vi "Test Harness.vi"(9 "Solver VI":refnum<vi>, 10 "Word List":string[](array[string])=["YELLOW", "ORANGE", "PURPLE", "BLUE", "GREEN", "RED"], 11 "Word Search Grid":string[][](array[string])=[["R", "B", "L", "U", "E", "W"], ["E", "G", "N", "A", "R", "O"], ["D", "B", "C", "E", "W", "L"], ["L", "L", "D", "K", "V", "L"], ["P", "U", "R", "P", "L", "E"], ["N", "E", "E", "R", "G", "Y"]]) -> (2 "All Words Found":bool, 3 "Execution Time":dbl)   [LabVIEW 2024]
panel:
  # "Use this Test Harness VI to time your Word Search solution (and ensure it works correctly)."
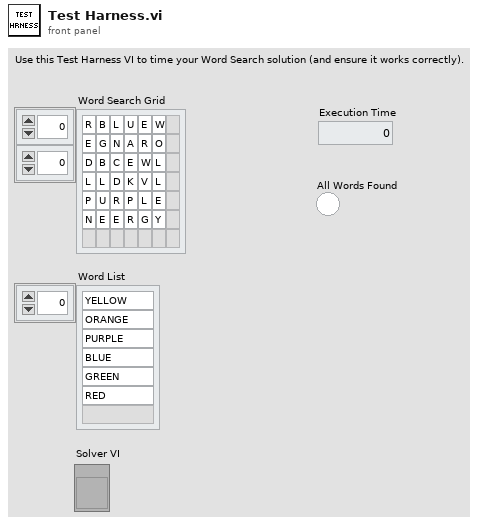
[diagram p1: front panel]
types:
  T1 = typedef "Word Search Scorer.lvlib/Solutions--map.ctl" = map{string, T2[]}
  T2 = typedef "Word Search Scorer.lvlib/Letter Index--cluster.ctl" = cluster{"Row":i32, "Column":i32}
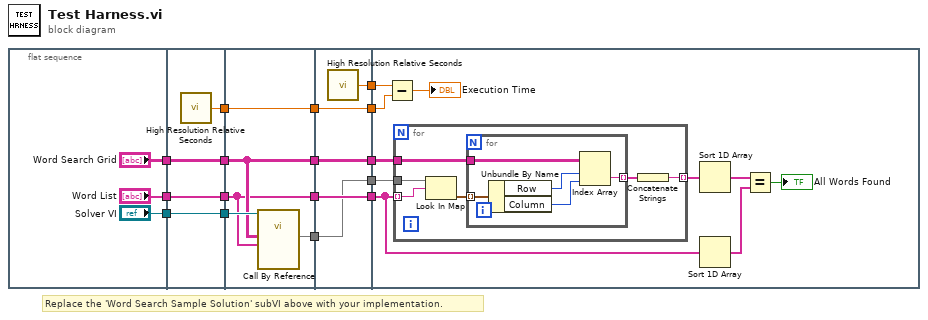
[diagram p0: block diagram]
diagram:
  # "Replace the 'Word Search Sample Solution' subVI above with your implementation."
  n1 = flat-sequence {
    tunnel: ["Word Search Grid"] -> w16
    tunnel: ["Word List"] -> w15
    tunnel: ["Solver VI"] -> w2
    tunnel: w16 -> [w21]
    tunnel: w15 -> [w23]
    tunnel: [w23] -> w14
    tunnel: [w22] -> w11
    tunnel: [w21] -> w4
    tunnel: [w20] -> w3
    tunnel: w2 -> [w20]
    tunnel: w14 -> [w25]
    tunnel: w11 -> [w28]
    tunnel: [w28] -> w10
    tunnel: [w25] -> w7
    tunnel: [w26] -> w5
    tunnel: w4 -> [w26]
    tunnel: w3 -> [w27]
    tunnel: [w24] -> w1
    tunnel: [w29] -> w13
    tunnel: [w33] -> w12
    tunnel: w10 -> [w32]
    tunnel: [w32] -> w9
    tunnel: [w31] -> w8
    tunnel: w7 -> [w31]
    tunnel: [w30] -> w6
    tunnel: w5 -> [w30]
    tunnel: w1 -> [w29]
    tunnel: w13 -> [w40]
    tunnel: w12 -> [w43]
    tunnel: w9 -> [w42]
    tunnel: w8 -> [w37]
    tunnel: w6 -> [w39]
    frame #0 {
    }
    frame #1 {
      n2 = call <vilib>:"High Resolution Relative Seconds.vi"() -> ("relative seconds"=w22:dbl)
    }
    frame #2 {
      n3 = call-by-ref "?"(reference=w27, "Word List"=w25, "Word Search Grid"=w26) -> ("Solutions"=w24:T1)  [unwired: 10 in, 2 out]
    }
    frame #3 {
      n4 = call <vilib>:"High Resolution Relative Seconds.vi"() -> ("relative seconds"=w33:dbl)
    }
    frame #4 {
      n5 = Subtract(x=w43, y=w42) -> (x-y=→"Execution Time":dbl)
      n6 = for {
        tunnel: w37 -> [w48] mode=indexing
        tunnel: w40 -> [w49]
        tunnel: w39 -> [w46]
        tunnel: [w44] -> w38 mode=indexing
        n7 = Look In Map(map=w49, key=w48) -> (value=w47:T2[])  [unwired: 1 in, 1 out]
        n8 = for {
          tunnel: w47 -> [w54] mode=indexing
          tunnel: w46 -> [w52]
          tunnel: [w50] -> w45 mode=indexing
          n9 = Unbundle By Name(w54) -> ("Row"=w53:i32, "Column"=w51:i32)
          n10 = Index Array(array=w52, index (row)=w53, index (col)=w51) -> (element=w50:string)
        }
        n11 = Concatenate Strings(w45) -> (w44:string)
      }
      n12 = Sort 1D Array(array=w38) -> (sorted array=w36:string[])
      n13 = Sort 1D Array(array=w37) -> (sorted array=w35:string[])
      n14 = Equal?(x=w36, y=w35) -> (x = y?=→"All Words Found":bool)
    }
  }
